vi "Calibr SpectraCalibration.vi"(8 "error in (no error)":errorcluster, 10 "Spectra in":cluster{"X":dbl[], "Y":dbl[]}[](array[cluster])) -> (0 "error out":errorcluster, 2 "Spectra out":cluster{"X":dbl[], "Y":dbl[]}[](array[cluster]))   [LabVIEW 2018, in "Calibr.lvclass"]
uses:
  Calibr.lvclass
  Calibr.lvclass/Calibr.ctl
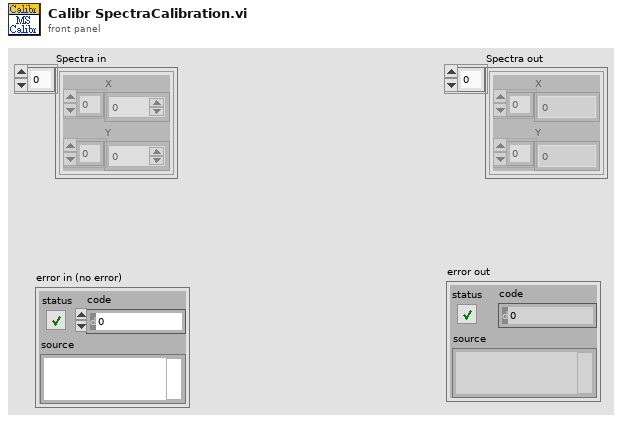
[diagram p1: front panel]
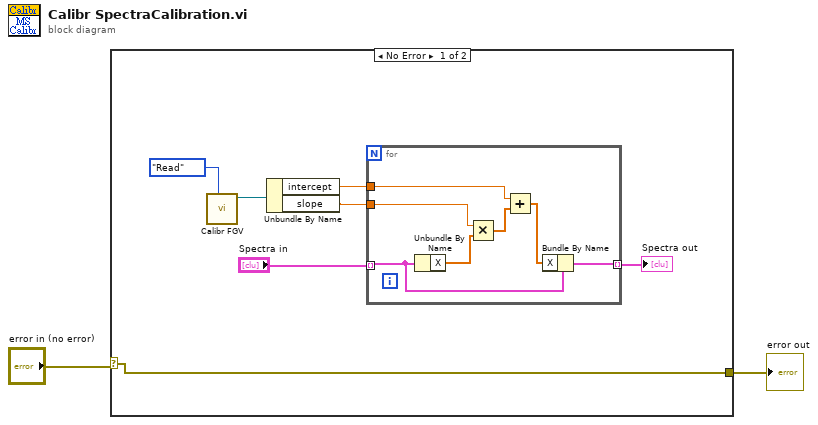
[diagram p0: block diagram]
diagram:
  n1 = case shown="No Error" "error in (no error)" {
    selector: "error in (no error)" -> [w3 w17]
    tunnel: [w3 w17] -> w1
    frame No Error {
      n2 = call "Calibr FGV.vi"("Function"=enum16{"Init", "Read", "Write"}."Read") -> ("Calibr out"=w8:refnum<class "Calibr.lvclass">)  [unwired: 9 in, 1 out]
      n3 = Unbundle By Name(w8) -> ("intercept"=w6:dbl, "slope"=w7:dbl)
      n4 = for {
        tunnel: w7 -> [w14]
        tunnel: w6 -> [w12]
        tunnel: "Spectra in" -> [w16] mode=indexing
        tunnel: [w10] -> w4 mode=indexing
        n5 = Unbundle By Name(w16) -> ("X"=w15:dbl[])
        n6 = Multiply(x=w14, y=w15) -> (x*y=w13:dbl[])
        n7 = Add(x=w12, y=w13) -> (x+y=w11:dbl[])
        n8 = Bundle By Name(cluster=w16, "X"=w11) -> (w10:cluster{"X":dbl[], "Y":dbl[]})
      }
      "Spectra out" <- w4
    }
    frame Error {
    }
  }
  "error out" <- w1
